vi "StartProcess.vi"(0 "reference in":refnum<class "ZeroMQ.lvclass">, 3 "ms timeout (-1)":i32=-1, 5 "error in (no error)":errorcluster) -> (14 "reference out":refnum<class "ZeroMQ.lvclass">, 15 "EventFromProcess":refnum<user-event>, 16 "timed out":bool, 19 "error out":errorcluster)   [LabVIEW 2018, in "ZeroMQ.lvclass"]
doc: "Looks up an existing object matching object name or creates a new object and returns a refnum you can use when calling other class methods.\n\nObjects created with this VI should be destroyed using this class Delete VI."
uses:
  ZeroMQ.lvclass
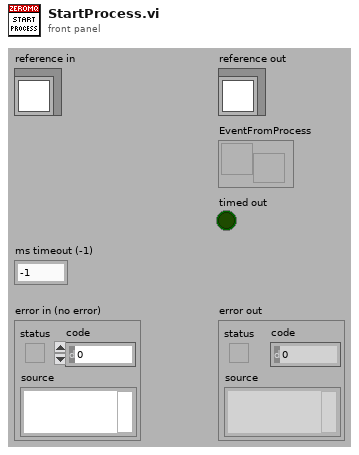
[diagram p1: front panel]
types:
  T1 = enum16{"ReadRepository", "CreateNew", "CreateOrLookUpExisting", "ReadRepositoryAndDestroy"}
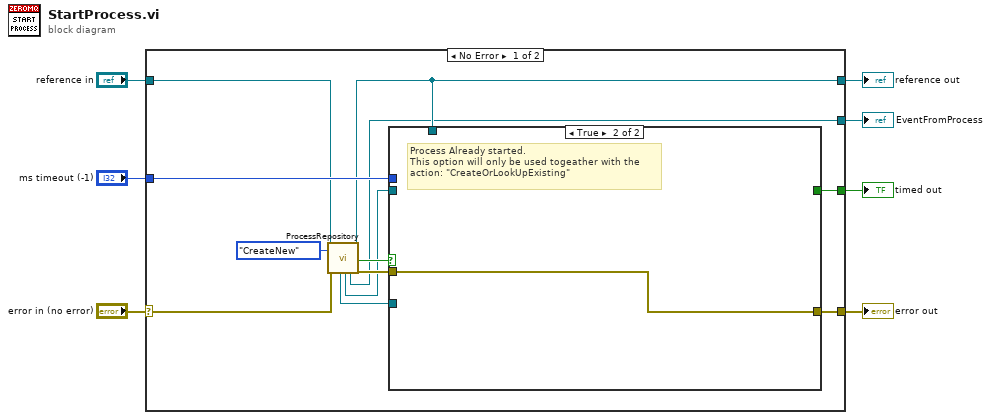
[diagram p0: block diagram]
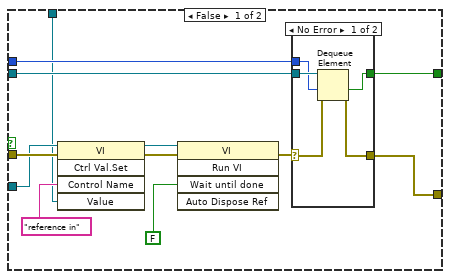
[diagram p2: hidden frame]
diagram:
  n1 = case shown="No Error" "error in (no error)" {
    selector: "error in (no error)" -> [w15 w39]
    tunnel: [w16 w39] -> w4
    tunnel: [w11 w40] -> w1
    tunnel: "reference in" -> [w10 w40]
    tunnel: "ms timeout (-1)" -> [w18 _]
    tunnel: [w17 _] -> w3
    tunnel: [w9 _] -> w2
    frame No Error {
      n2 = call "ProcessRepository.vi"("reference in"=w10, "Action(ReadRepository)"=T1."CreateNew", "error in (no error)"=w15) -> ("ProcessViRef"=w13:refnum<vi>, "ProcessSyncQueue"=w12:refnum<queue>, "EventFromProcess"=w9:refnum<user-event>, "reference out"=w11:refnum<class "ZeroMQ.lvclass">, "ProcessAlreadyStarted"=w19:bool, "error out"=w14:errorcluster)  [unwired: 9 in, 2 out]
      n3 = case shown="True" w19 {
        tunnel: w18 -> [w27 _]
        tunnel: [w26 _] -> w17
        tunnel: [w24 w38] -> w16
        tunnel: w14 -> [w23 w38]
        tunnel: w13 -> [w22 _]
        tunnel: w12 -> [w21 _]
        tunnel: w11 -> [w20 _]
        frame False {
          n4 = invoke class="VI" method="Ctrl Val.Set"(reference=w22, error in=w23, "Control Name"="reference in", "Value"=w20) -> (reference out=w30:refnum<vi>, error out=w29:errorcluster)  [unwired: 1 in, 3 out]
          n5 = invoke class="VI" method="Run VI"(reference=w30, error in=w29, "Wait until done"=FALSE ("Wait Until Done")) -> (error out=w25:errorcluster)  [unwired: 2 in, 4 out]
          n6 = case shown="No Error" w25 {
            tunnel: w21 -> [w36 _]
            tunnel: w27 -> [w32 _]
            tunnel: [w33 _] -> w26
            selector: w25 -> [w35 w37]
            tunnel: [w34 w37] -> w24
            frame No Error {
              n7 = Dequeue Element(queue=w36, timeout in ms (-1)=w32, error in (no error)=w35) -> (timed out?=w33:bool, error out=w34:errorcluster)  [unwired: 2 out]
            }
            frame Error {
            }
          }
        }
        frame True {
          # "Process Already started.\nThis option will only be used togeather with the\naction: \"CreateOrLookUpExisting\""
        }
      }
    }
    frame Error {
    }
  }
  "error out" <- w4
  "reference out" <- w1
  "timed out" <- w3
  "EventFromProcess" <- w2
